vi "XML_Deserialize_XML_File_Error_Handling.vi"(8 "error in (no error)":errorcluster) -> (0 "error out":errorcluster)   [LabVIEW 2013, in "XML_Deserializer.lvlib"]
uses:
  XML_Deserializer.lvlib
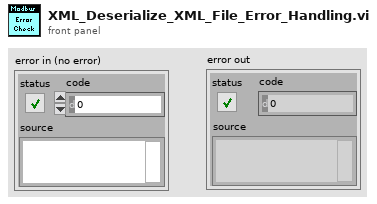
[diagram p1: front panel]
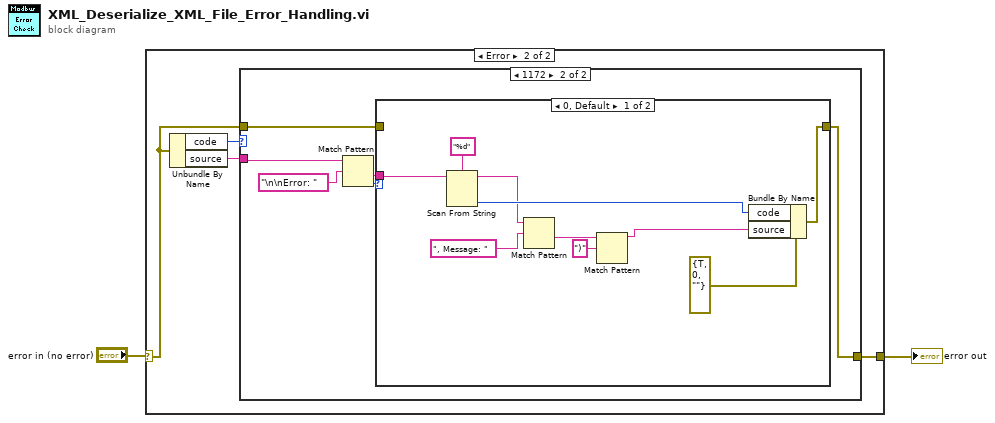
[diagram p0: block diagram]
diagram:
  n1 = case shown="Error" "error in (no error)" {
    selector: "error in (no error)" -> [w3 w5]
    tunnel: [w3 w4] -> w1
    frame No Error {
    }
    frame Error {
      n2 = Unbundle By Name(w5) -> ("code"=w7:i32, "source"=w6:string)
      n3 = case shown="1172" w7 {
        tunnel: w6 -> [_ w14]
        tunnel: w5 -> [w8 w11]
        tunnel: [w8 w10] -> w4
        frame 0, Default {
        }
        frame 1172 {
          n4 = Match Pattern(string=w14, regular expression="\n\nError: " ("format string")) -> (after substring=w9:string, offset past match=w12:i32)  [unwired: 1 in, 2 out]
          n5 = case shown="0, Default" w12 {
            tunnel: w11 -> [_ w25]
            tunnel: [w20 w25] -> w10
            tunnel: w9 -> [w24 _]
            frame 0, Default {
              n6 = Scan From String(format string="%d", input string=w24) -> (remaining string=w19:string, output 1=w21:i32)  [unwired: 3 in, 2 out]
              n7 = Match Pattern(string=w19, regular expression=", Message: " ("format string")) -> (after substring=w17:string)  [unwired: 1 in, 3 out]
              n8 = Match Pattern(string=w17, regular expression=")") -> (before substring=w15:string)  [unwired: 1 in, 3 out]
              n9 = Bundle By Name(cluster=errorcluster {"status"=TRUE, "code"=0, "source"=""} ("error IO"), "code"=w21, "source"=w15) -> (w20:errorcluster)
            }
            frame -1 {
            }
          }
        }
      }
    }
  }
  "error out" <- w1
